vi "Generate 16ms Pulse and Test AC Rise Time V2.vi"(0 "Device Name":string="Dev2", 1 "offset":dbl=1.25, 3 "#Samples":i32=48000, 5 "rate":dbl=600000.0, 9 "frequency":dbl=62.5, 12 "square wave \nduty cycle (%)":dbl=50.0, 13 "nWhichChan":i32=1, 14 "amplitude (pk)":dbl=1.25) -> (6 "Return Code":i32, 15 "error out":errorcluster)   [LabVIEW 2015]
doc: "This VI generates the square wave 62.5Hz, duty cycle 50%, 2.5V pk, 0VDC offset and perform\nthe AC rise test using TestAnalogFrontEnd dll function call.\n\nint nWhichChan – integer value with which channel to test (values 1 –4).\n\nThis function returns a 0 if the function completed successfully. A non-zero return code will indicate error."
uses:
  <vilib>/DAQmx/write.llb/DAQmx Write (Analog 1D Wfm NChan NSamp).vi
  <vilib>/DAQmx/create/channels.llb/DAQmx Create Channel (AO-Voltage-Basic).vi
  <vilib>/DAQmx/configure/timing.llb/DAQmx Timing (Sample Clock).vi
  <vilib>/DAQmx/miscellaneous.llb/DAQmx Fill In Error Info.vi
  <resource>/objmgr/daqmx.rc
  <vilib>/measure/NI_MABase.lvlib
panel:
  out "Waveform Graph":waveform(dbl)(graph)={"t0"=timestamp(0 s since 1904-01-01), "dt"=1.25e-06, "Y"=array[64000 elements]}
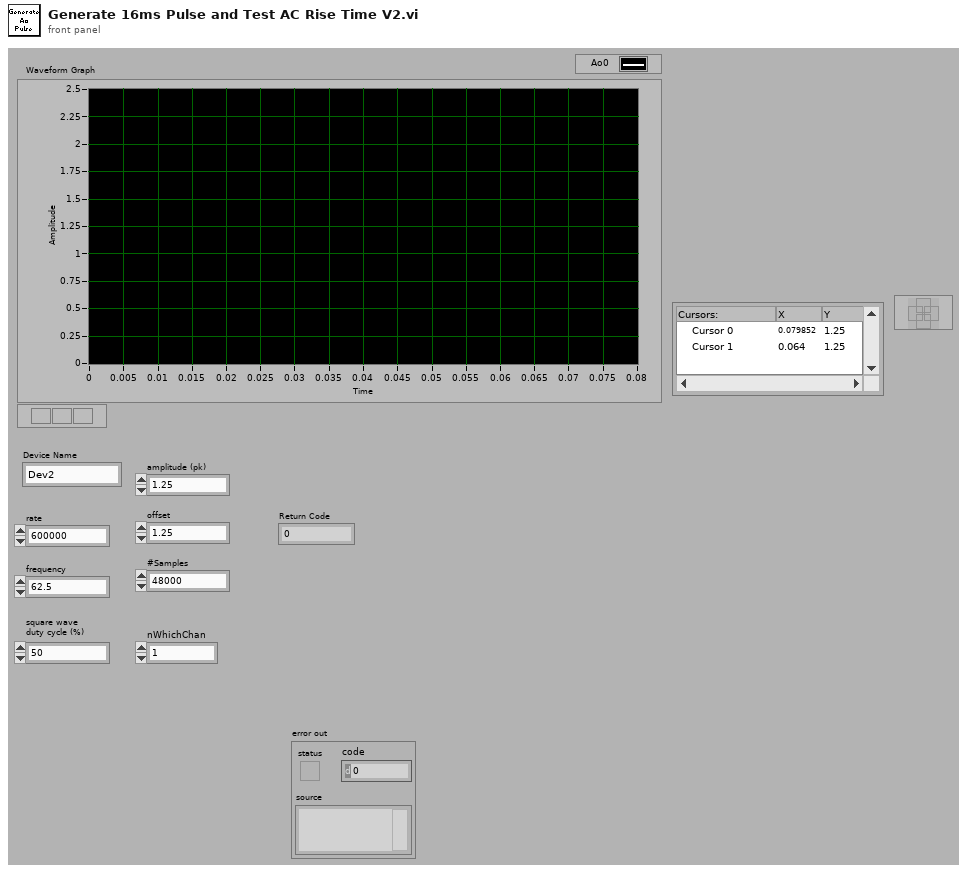
[diagram p1: front panel]
types:
  T1 = enum16{"Sine Wave", "Triangle Wave", "Square Wave", "Sawtooth Wave"}
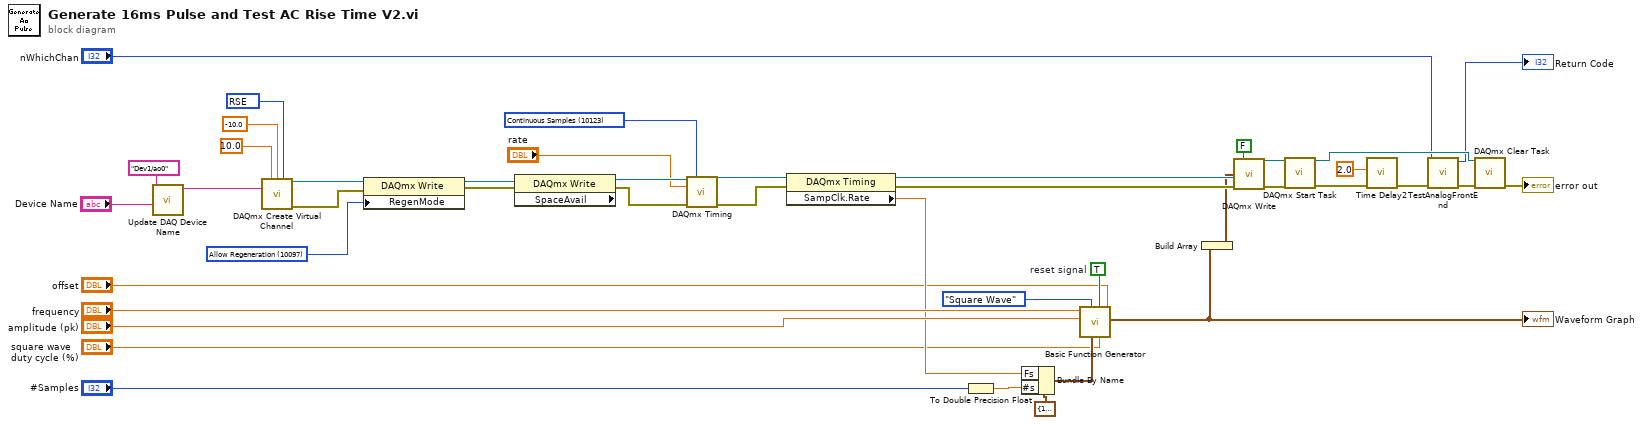
[diagram p0: block diagram]
diagram:
  w11 = 10123 items=["Finite Samples"=10178, "Continuous Samples"=10123, "Hardware Timed Single Point"=12522] ("sample mode")
  w14 = 10083 items=["Default"=-1, "RSE"=10083, "Differential"=10106, "Pseudodifferential"=12529] ("output terminal configuration")
  w26 = TRUE  # reset signal
  w41 = 10097 items=["Allow Regeneration"=10097, "Do Not Allow Regeneration"=10158] ("RegenMode")
  n1 = call "Update DAQ Device Name.vi"("Device Name"="Device Name", "Lines in (String)"="Dev1/ao0" ("Channel names")) -> ("Lines out"=w4:tag)  [unwired: 9 in]
  n2 = call-poly <vilib>:"DAQmx Create Virtual Channel.vi"("maximum value"=10.0, "minimum value"=-10.0, "output terminal configuration"=w14, "physical channels"=w4) -> ("task out"=w43:refnum<k21>, "error out"=w42:errorcluster)  [unwired: 10 in]
  n3 = property class="DAQmx Write"(reference=w43, error in=w42, "RegenMode"=w41) -> (reference out=w39:refnum<k21>, error out=w40:errorcluster)
  n4 = property class="DAQmx Write" props=["SpaceAvail"](reference=w39, error in=w40) -> (reference out=w38:refnum<k21>, error out=w37:errorcluster)  [unwired: 1 out]
  n5 = call-poly <vilib>:"DAQmx Timing.vi"("task/channels in"=w38, "sample mode"=w11, "rate"="rate", "error in"=w37) -> ("task out"=w36:refnum<k21>, "error out"=w35:errorcluster)  [unwired: 10 in]
  n6 = property class="DAQmx Timing"(reference=w36, error in=w35) -> (reference out=w19:refnum<k21>, error out=w20:errorcluster, "SampClk.Rate"=w29:dbl)
  n7 = To Double Precision Float(number="#Samples") -> (double precision float=w28:dbl)
  n8 = Bundle By Name(cluster=cluster{"Fs":dbl, "#s":dbl} {"Fs"=1000.0, "#s"=1000.0} ("sampling info"), "Fs"=w29, "#s"=w28) -> (w31:cluster{"Fs":dbl, "#s":dbl})
  n9 = call <vilib>:"Basic Function Generator.vi"("offset"="offset", "square wave duty cycle (%)"="square wave \nduty cycle (%)", "reset signal"=w26, "sampling info"=w31, "signal type"=T1."Square Wave", "amplitude"="amplitude (pk)", "frequency"="frequency") -> ("signal out"=w12:waveform(dbl))  [unwired: 2 in, 2 out]
  "Waveform Graph" <- w12
  n10 = Build Array(w12) -> (w13:waveform(dbl)[])
  n11 = call-poly <vilib>:"DAQmx Write.vi"("task/channels in"=w19, "auto start"=FALSE, "data"=w13, "error in"=w20) -> ("task out"=w17:refnum<k21>, "error out"=w18:errorcluster)  [unwired: 9 in, 1 out]
  n12 = call <vilib>:"DAQmx Start Task.vi"("task/channels in"=w17, "error in"=w18) -> ("task out"=w10:refnum<k21>, "error out"=w6:errorcluster)  [unwired: 12 in]
  n13 = call "Time Delay2"("error in (no error)"=w6, "Delay Time (s)"=2.0) -> ("error out"=w5:errorcluster)  [unwired: 9 in]
  n14 = call "TestAnalogFrontEnd.vi"("error in"=w5, "nWhichChan"="nWhichChan") -> ("error out"=w9:errorcluster, "Return Code"=→"Return Code":i32)  [unwired: 8 in]
  n15 = call <vilib>:"DAQmx Clear Task.vi"("task in"=w10, "error in"=w9) -> ("error out"=→"error out":errorcluster)  [unwired: 13 in]
